vi "Clean Output Terminal Label.vi"(8 "error in (no error)":errorcluster, 11 "control in":refnum<vi>) -> (0 "error out":errorcluster, 3 "control out":refnum<vi>)   [LabVIEW 2017]
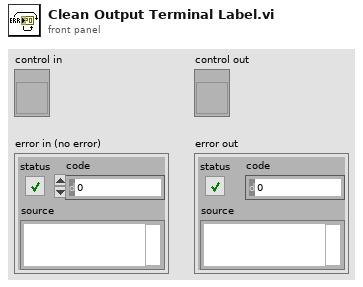
[diagram p1: front panel]
types:
  T1 = typedef "LVRectTypeDef.ctl" = cluster{"Left":i16, "Top":i16, "Right":i16, "Bottom":i16}
  T2 = cluster{"Left":i32, "Top":i32, "Right":i32, "Bottom":i32}
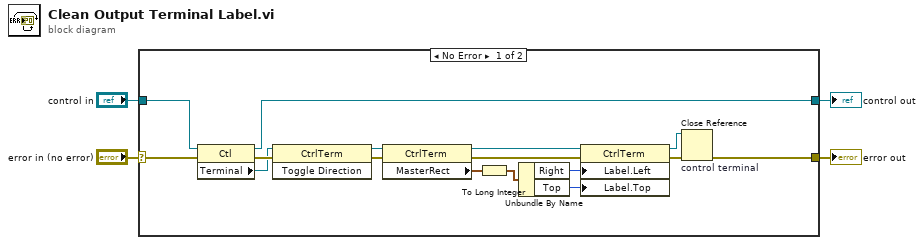
[diagram p0: block diagram]
diagram:
  n1 = case shown="No Error" "error in (no error)" {
    selector: "error in (no error)" -> [w5 w21]
    tunnel: "control in" -> [w15 w22]
    tunnel: [w9 w22] -> w3
    tunnel: [w7 w21] -> w2
    frame No Error {
      n2 = property class="Ctl"(reference=w15, error in=w5) -> (reference out=w9:refnum<vi>, error out=w14:errorcluster, "Terminal"=w10:refnum<vi>)
      n3 = invoke class="CtrlTerm" method="Toggle Direction"(reference=w10, error in=w14) -> (reference out=w13:refnum<vi>, error out=w11:errorcluster)  [unwired: 1 in, 1 out]
      n4 = property class="CtrlTerm"(reference=w13, error in=w11) -> (reference out=w16:refnum<vi>, error out=w17:errorcluster, "MasterRect"=w20:T1)
      n5 = To Long Integer(number=w20) -> (32bit integer=w12:T2)
      n6 = Unbundle By Name(w12) -> ("Right"=w19:i32, "Top"=w18:i32)
      n7 = property class="CtrlTerm"(reference=w16, error in=w17, "Label.Left"=w19, "Label.Top"=w18) -> (reference out=w6:refnum<vi>, error out=w8:errorcluster)
      n8 = Close Reference "control terminal"(reference=w6, error in (no error)=w8) -> (error out=w7:errorcluster)
    }
    frame Error {
    }
  }
  "control out" <- w3
  "error out" <- w2
